vi "KE6221 -- Set Output State.vi"(0 "Resource In":refnum<visa-resource-name>, 1 "Check For SCPI Errors? (T)":bool=TRUE, 7 "Output State":T1, 11 "error in (no error)":errorcluster) -> (4 "Resource Out (dupl)":refnum<visa-resource-name>, 15 "error out":errorcluster)   [LabVIEW 2013, in "Keithly user program.lvlib"]
doc: "Sets the output state of the 622x current source, either 'On' or 'Off'."
uses:
  Keithly user program.lvlib
  Typedefs/KE622x -- On Off Control.ctl
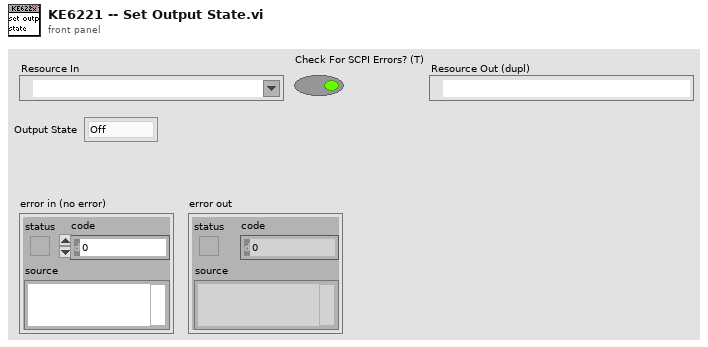
[diagram p1: front panel]
types:
  T1 = typedef "Keithly user program.lvlib/KE622x -- On Off Control.ctl" = enum16{"Off", "On"}
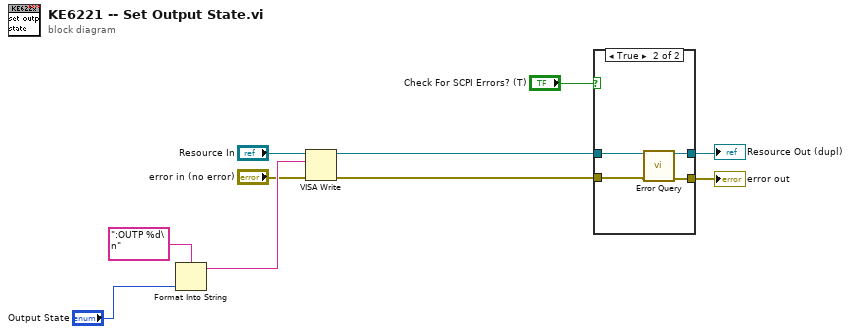
[diagram p0: block diagram]
diagram:
  n1 = Format Into String(format string=":OUTP %d\n", "Output State") -> (resulting string=w8:string)  [unwired: 2 in, 1 out]
  n2 = VISA Write(VISA resource name="Resource In", write buffer=w8, error in (no error)="error in (no error)") -> (VISA resource name out=w5:refnum<visa-resource-name>, error out=w4:errorcluster)  [unwired: 1 out]
  n3 = case shown="True" "Check For SCPI Errors? (T)" {
    tunnel: w5 -> [w12 w15]
    tunnel: w4 -> [w11 w14]
    tunnel: [w11 w13] -> w2
    tunnel: [w12 w16] -> w3
    frame False {
    }
    frame True {
      n4 = call "Error Query.vi"("VISA Resource In"=w15, "error in (no error)"=w14) -> ("VISA Resource Out (dupl)"=w16:refnum<visa-resource-name>, "error out"=w13:errorcluster)  [unwired: 10 in, 2 out]
    }
  }
  "Resource Out (dupl)" <- w3
  "error out" <- w2
